vi "ReadTree.vi"(8 "error in":errorcluster, 10 "root":T1, 11 "CEF_Repository in":refnum<class "CEF_Repository.lvclass">) -> (0 "error out":errorcluster, 3 "CEF_Repository out":refnum<class "CEF_Repository.lvclass">)   [LabVIEW 2023, in "CEF.lvlib" / "CEF_Repository.lvclass"]
doc: "Transfers information between the repo and the tree control nodes. This should be called before custom views are launched or saving to disk.Copyright 2017 National Instruments Corporation\n\nLicensed under the Apache License, Version 2.0 (the \"License\"); you may not use this file except in compliance with the License. You may obtain a copy of the License at http://www.apache.org/licenses/LICENSE-2.0\nUnless required by applicable law or agreed to in writing, software distributed under the License is distributed on an \"AS IS\" BASIS, WITHOUT WARRANTIES OR CONDITIONS OF ANY KIND, either express or implied. See the License for the specific language governing permissions and limitations under the License."
uses:
  CEF_Repository.lvclass
  Node/NodeRef.ctl
  Node/CEF_Node.lvclass
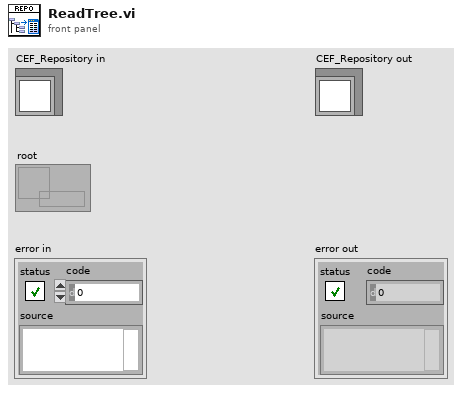
[diagram p1: front panel]
types:
  T1 = typedef "CEF.lvlib/CEF_Node.lvclass/NodeRef.ctl" = refnum<data-value>
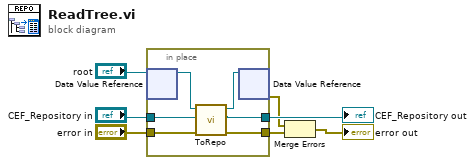
[diagram p0: block diagram]
diagram:
  n1 = in-place {
    in-place-border: "error in" -> [w11]
    in-place-border: [w10] -> w2
    in-place-border: "CEF_Repository in" -> [w9]
    in-place-border: [w8] -> w4
    n2 = in-place-dvr #1("root") -> (w13:refnum<class "CEF_Node.lvclass">)  [unwired: 1 out]
    n3 = call-dynamic "ToRepo.vi"("error in"=w11, "repository in"=w9, "CEF_Node in"=w13) -> ("error out"=w10:errorcluster, "repository out"=w8:refnum<class "CEF_Repository.lvclass">, "CEF_Node out"=w12:refnum<class "CEF_Node.lvclass">)  [unwired: 6 in]
    n4 = in-place-dvr #1(w12) -> (w1:errorcluster)  [unwired: 1 out]
  }
  "CEF_Repository out" <- w4
  n5 = Merge Errors(w1, w2) -> (→"error out":errorcluster)
